vi "Autobalance Calculate One DOF.vi"(6 "Max Voltage":dbl, 8 "Autobalance Persistant Values In":T1, 10 "Error Tolerance":dbl) -> (0 "Autobalance Persistant Values Out":T1, 2 "Balanced Command":dbl)   [LabVIEW 2009]
uses:
  Autobalance Status Data.ctl
  Apps/Yes No Button.ctl
  Autobalance Stage.ctl
  Autobalance Data Point.ctl
  Course2MediumTransition.ctl
panel:
  # "Cmd"
  # "Servo"
  # "Cmd"
  # "Servo"
  # "Cmd"
  # "Servo"
  # "Cmd"
  # "Servo"
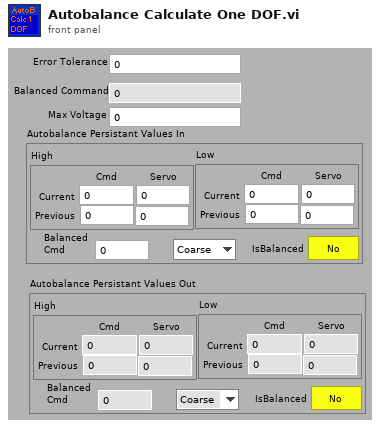
[diagram p1: front panel]
types:
  T1 = typedef "Autobalance Status Data.ctl" = cluster{"IsBalanced":T2, "Autobalance Stage":T3, "High":T4, "Low":T4, "Balanced \nCmd":dbl}
  T2 = typedef "Yes No Button.ctl" = bool
  T3 = typedef "Autobalance Stage.ctl" = enum16{"Coarse", "Fine", "Done"}
  T4 = typedef "Autobalance Data Point.ctl" = cluster{"cCmd":dbl, "cServo":dbl, "pCmd":dbl, "pServo":dbl}
  T5 = typedef "Course2MediumTransition.ctl" = enum16{"High Changed", "Low Changed", "Both Changed", "None Changed"}
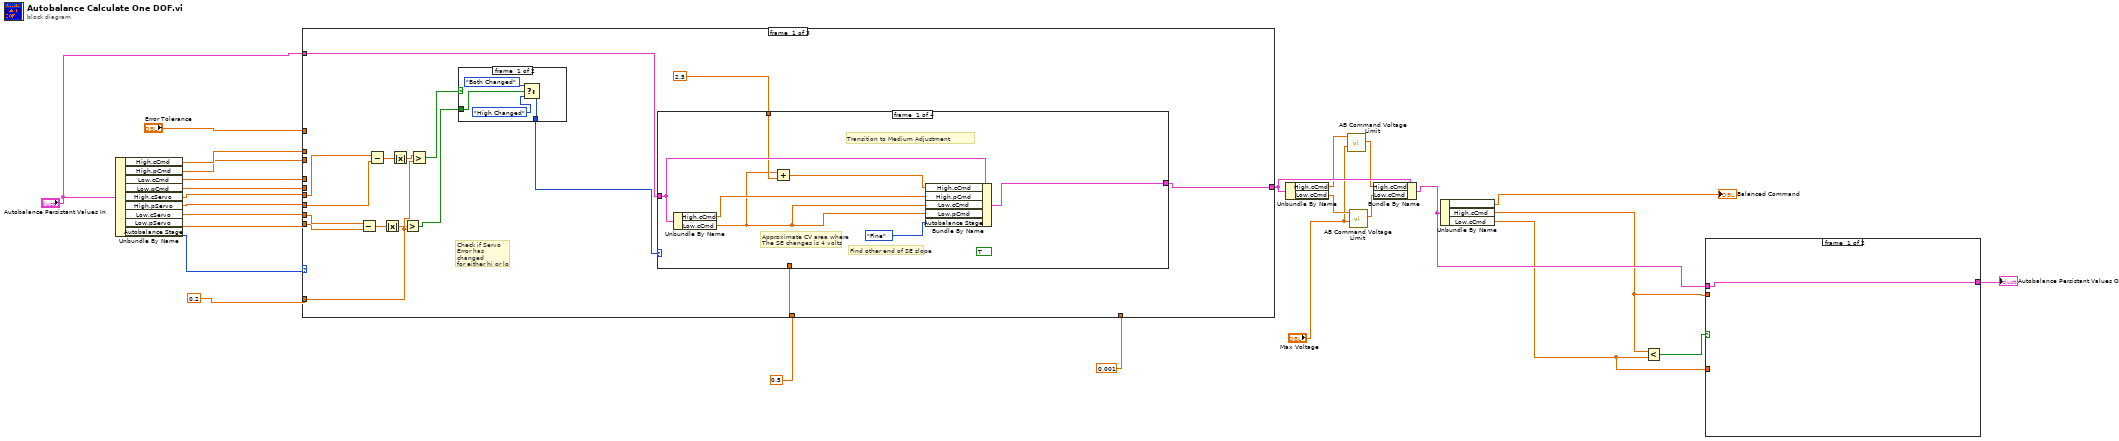
[diagram p0: block diagram]
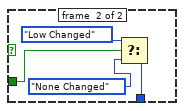
[diagram p2: hidden frame]
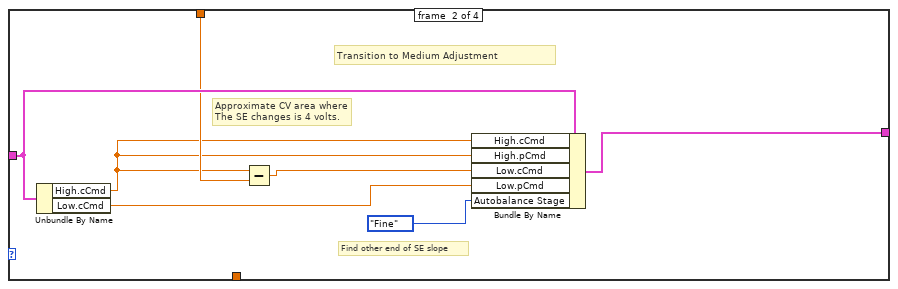
[diagram p3: hidden frame]
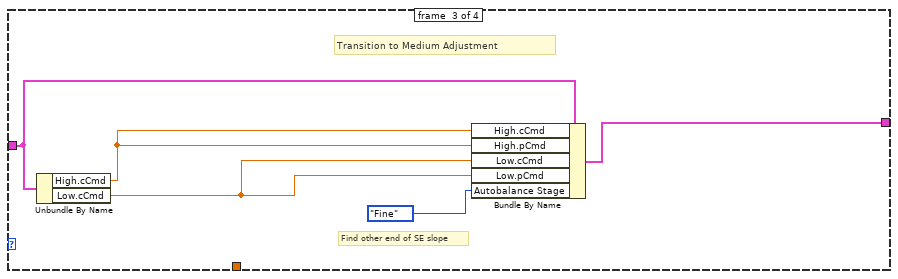
[diagram p4: hidden frame]
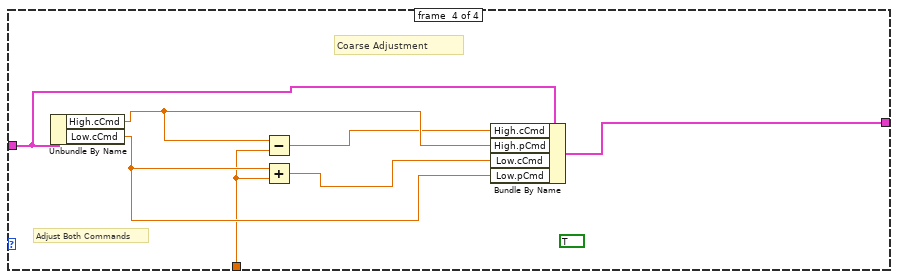
[diagram p5: hidden frame]
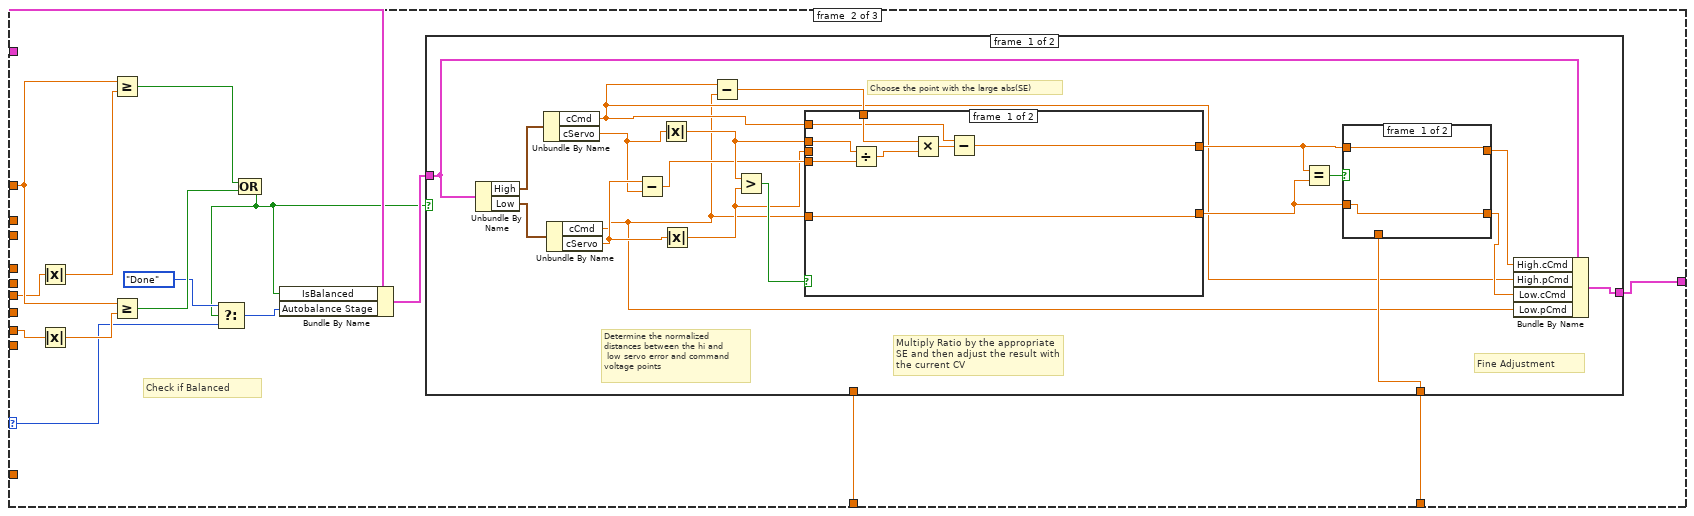
[diagram p6: hidden frame]
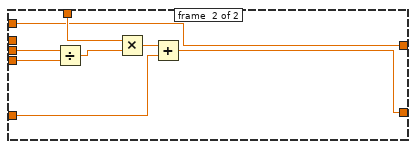
[diagram p7: hidden frame]
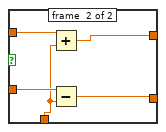
[diagram p8: hidden frame]
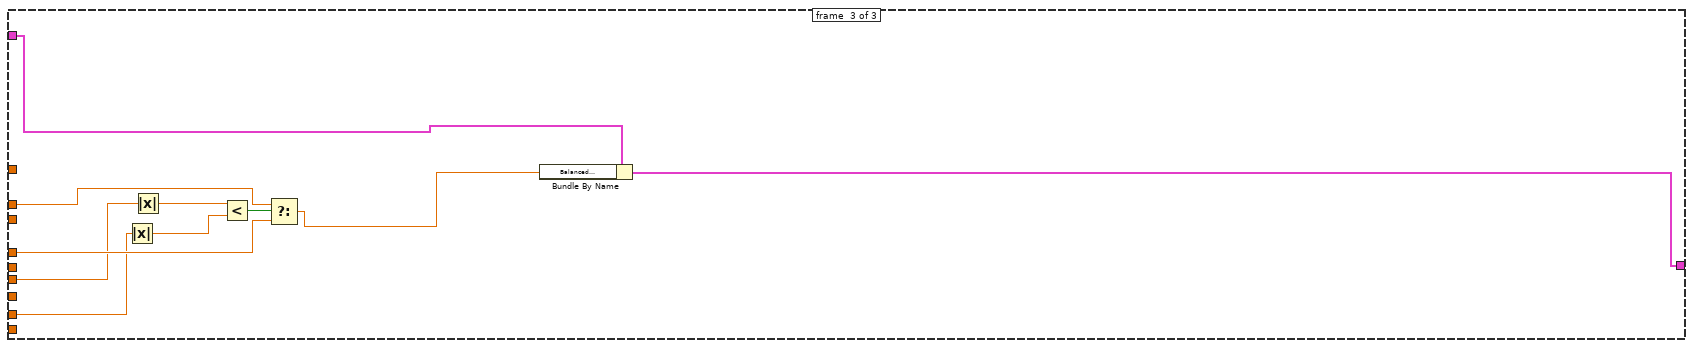
[diagram p10: hidden frame]
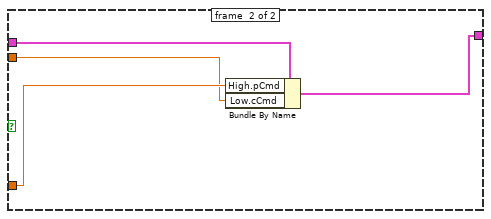
[diagram p11: hidden frame]
diagram:
  n1 = Unbundle By Name("Autobalance Persistant Values In") -> ("High.cCmd"=w17:dbl, "High.pCmd"=w16:dbl, "Low.cCmd"=w15:dbl, "Low.pCmd"=w14:dbl, "High.cServo"=w26:dbl, "High.pServo"=w25:dbl, "Low.cServo"=w24:dbl, "Low.pServo"=w23:dbl, "Autobalance Stage"=w22:T3)
  n2 = case shown="\"Fine\"" w22 {
    selector: w22 -> [_ w87 _]
    tunnel: w26 -> [w41 w81 w140]
    tunnel: w25 -> [w42 _ _]
    tunnel: w24 -> [w40 w80 w139]
    tunnel: w23 -> [w39 _ _]
    tunnel: "Autobalance Persistant Values In" -> [w28 w88 w138]
    tunnel: [w36 w83 w136] -> w6
    tunnel: "Error Tolerance" -> [_ w85 _]
    tunnel: 0.2 -> [w38 _ _]
    tunnel: 0.5 -> [w37 w78 _]
    tunnel: w17 -> [_ _ w142]
    tunnel: w16 -> [_ _ _]
    tunnel: w15 -> [_ _ w141]
    tunnel: w14 -> [_ _ _]
    tunnel: 0.001 -> [_ w77 _]
    frame #0 {
      # "Check if Servo \nError has changed\nfor either hi or lo"
      n3 = Subtract(x=w40, y=w39) -> (x-y=w33:dbl)
      n4 = Subtract(x=w41, y=w42) -> (x-y=w35:dbl)
      n5 = Absolute Value(x=w33) -> (abs(x)=w32:dbl)
      n6 = Absolute Value(x=w35) -> (abs(x)=w34:dbl)
      n7 = Greater?(x=w32, y=w38) -> (0:w30:bool)
      n8 = Greater?(x=w34, y=w38) -> (0:w31:bool)
      n9 = case shown="True" w31 {
        tunnel: w30 -> [w46 w50]
        tunnel: [w43 w47] -> w29
        frame #0 {
          n10 = Select(t=Course2MediumTransition."Both Changed", s=w46, f=Course2MediumTransition."High Changed" ("Course2MediumTransition")) -> (s? t:f=w43:T5)
        }
        frame #1 {
          n11 = Select(t=Course2MediumTransition."Low Changed", s=w50, f=Course2MediumTransition."None Changed" ("Course2MediumTransition")) -> (s? t:f=w47:T5)
        }
      }
      n12 = case shown="\"High Changed\"" w29 {
        tunnel: w28 -> [w57 w64 w69 w76]
        tunnel: [w56 w63 w68 w75] -> w36
        tunnel: w37 -> [_ _ _ w72]
        tunnel: 2.5 -> [w54 w59 _ _]
        frame #0 {
          (unwired) TRUE
          # "Approximate CV area where\nThe SE changes is 4 volts"
          # "Transition to Medium Adjustment"
          # "Find other end of SE slope"
          n13 = Unbundle By Name(w57) -> ("High.cCmd"=w53:dbl, "Low.cCmd"=w51:dbl)
          n14 = Add(x=w51, y=w54) -> (x+y=w52:dbl)
          n15 = Bundle By Name(cluster=w57, "High.cCmd"=w52, "High.pCmd"=w53, "Low.cCmd"=w51, "Low.pCmd"=w51, "Autobalance Stage"=Autobalance_Stage."Fine" ("t")) -> (w56:T1)
        }
        frame #1 {
          # "Approximate CV area where\nThe SE changes is 4 volts."
          # "Transition to Medium Adjustment"
          # "Find other end of SE slope"
          n16 = Unbundle By Name(w64) -> ("High.cCmd"=w58:dbl, "Low.cCmd"=w61:dbl)
          n17 = Subtract(x=w58, y=w59) -> (x-y=w60:dbl)
          n18 = Bundle By Name(cluster=w64, "High.cCmd"=w58, "High.pCmd"=w58, "Low.cCmd"=w60, "Low.pCmd"=w61, "Autobalance Stage"=Autobalance_Stage."Fine" ("t")) -> (w63:T1)
        }
        frame #2 {
          # "Transition to Medium Adjustment"
          # "Find other end of SE slope"
          n19 = Unbundle By Name(w69) -> ("High.cCmd"=w66:dbl, "Low.cCmd"=w65:dbl)
          n20 = Bundle By Name(cluster=w69, "High.cCmd"=w66, "High.pCmd"=w66, "Low.cCmd"=w65, "Low.pCmd"=w65, "Autobalance Stage"=Autobalance_Stage."Fine" ("t")) -> (w68:T1)
        }
        frame #3 {
          (unwired) TRUE
          # "Coarse Adjustment"
          # "Adjust Both Commands"
          n21 = Unbundle By Name(w76) -> ("High.cCmd"=w74:dbl, "Low.cCmd"=w73:dbl)
          n22 = Subtract(x=w74, y=w72) -> (x-y=w71:dbl)
          n23 = Add(x=w73, y=w72) -> (x+y=w70:dbl)
          n24 = Bundle By Name(cluster=w76, "High.cCmd"=w71, "High.pCmd"=w74, "Low.cCmd"=w70, "Low.pCmd"=w73) -> (w75:T1)
        }
      }
    }
    frame #1 {
      # "Check if Balanced"
      n25 = Absolute Value(x=w81) -> (abs(x)=w89:dbl)
      n26 = Absolute Value(x=w80) -> (abs(x)=w90:dbl)
      n27 = Greater Or Equal?(x=w85, y=w89) -> (x >= y?=w91:bool)
      n28 = Greater Or Equal?(x=w85, y=w90) -> (x >= y?=w92:bool)
      n29 = Compound Arithmetic op=OR(w91, w92) -> (w82:bool)
      n30 = Select(t=Autobalance_Stage."Done", s=w82, f=w87) -> (s? t:f=w79:T3)
      n31 = Bundle By Name(cluster=w88, "IsBalanced"=w82, "Autobalance Stage"=w79) -> (w84:T1)
      n32 = case shown="False" w82 {
        tunnel: w84 -> [w109 w135]
        tunnel: [w108 w135] -> w83
        tunnel: w78 -> [_ _]
        tunnel: w77 -> [w106 _]
        frame #0 {
          # "Choose the point with the large abs(SE)"
          # "Multiply Ratio by the appropriate\nSE and then adjust the result with \nthe current CV"
          # "Determine the normalized \ndistances between the hi and\n low servo error and command\nvoltage points"
          # "Fine Adjustment"
          n33 = Unbundle By Name(w109) -> ("High"=w111:T4, "Low"=w110:T4)
          n34 = Unbundle By Name(w111) -> ("cCmd"=w94:dbl, "cServo"=w102:dbl)
          n35 = Unbundle By Name(w110) -> ("cCmd"=w93:dbl, "cServo"=w103:dbl)
          n36 = Subtract(x=w103, y=w102) -> (x-y=w99:dbl)
          n37 = Absolute Value(x=w102) -> (abs(x)=w100:dbl)
          n38 = Absolute Value(x=w103) -> (abs(x)=w95:dbl)
          n39 = Subtract(x=w94, y=w93) -> (x-y=w98:dbl)
          n40 = Greater?(x=w100, y=w95) -> (0:w101:bool)
          n41 = case shown="True" w101 {
            tunnel: w100 -> [w119 _]
            tunnel: w99 -> [w118 w127]
            tunnel: w98 -> [w116 w125]
            tunnel: w93 -> [w115 w123]
            tunnel: [w115 w120] -> w97
            tunnel: [w114 w121] -> w96
            tunnel: w95 -> [_ w122]
            tunnel: w94 -> [w112 w121]
            frame #0 {
              n42 = Divide(x=w119, y=w118) -> (x/y=w117:dbl)
              n43 = Multiply(x=w116, y=w117) -> (x*y=w113:dbl)
              n44 = Subtract(x=w112, y=w113) -> (x-y=w114:dbl)
            }
            frame #1 {
              n45 = Divide(x=w122, y=w127) -> (x/y=w126:dbl)
              n46 = Multiply(x=w125, y=w126) -> (x*y=w124:dbl)
              n47 = Add(x=w124, y=w123) -> (x+y=w120:dbl)
            }
          }
          n48 = Equal?(x=w96, y=w97) -> (x = y?=w107:bool)
          n49 = case shown="True" w107 {
            tunnel: w96 -> [w129 w132]
            tunnel: w97 -> [w128 w134]
            tunnel: w106 -> [_ w133]
            tunnel: [w129 w131] -> w105
            tunnel: [w128 w130] -> w104
            frame #0 {
            }
            frame #1 {
              n50 = Add(x=w132, y=w133) -> (x+y=w131:dbl)
              n51 = Subtract(x=w134, y=w133) -> (x-y=w130:dbl)
            }
          }
          n52 = Bundle By Name(cluster=w109, "High.cCmd"=w105, "High.pCmd"=w94, "Low.cCmd"=w104, "Low.pCmd"=w93) -> (w108:T1)
        }
        frame #1 {
        }
      }
    }
    frame #2 {
      n53 = Absolute Value(x=w139) -> (abs(x)=w144:dbl)
      n54 = Absolute Value(x=w140) -> (abs(x)=w143:dbl)
      n55 = Less?(x=w143, y=w144) -> (x < y?=w145:bool)
      n56 = Select(t=w142, s=w145, f=w141) -> (s? t:f=w137:dbl)
      n57 = Bundle By Name(cluster=w138, "Balanced \nCmd"=w137) -> (w136:T1)
    }
  }
  n58 = Unbundle By Name(w6) -> ("High.cCmd"=w5:dbl, "Low.cCmd"=w3:dbl)
  n59 = call "AB Command Voltage Limit.vi"("Max Voltage"="Max Voltage", "Command In"=w5) -> ("Command Out"=w4:dbl)  [unwired: 9 out]
  n60 = call "AB Command Voltage Limit.vi"("Max Voltage"="Max Voltage", "Command In"=w3) -> ("Command Out"=w2:dbl)  [unwired: 9 out]
  n61 = Bundle By Name(cluster=w6, "High.cCmd"=w4, "Low.cCmd"=w2) -> (w12:T1)
  n62 = Unbundle By Name(w12) -> ("Balanced \nCmd"=→"Balanced Command":dbl, "High.cCmd"=w11:dbl, "Low.cCmd"=w10:dbl)
  n63 = Less?(x=w11, y=w10) -> (x < y?=w13:bool)
  n64 = case shown="True" w13 {
    tunnel: w12 -> [w146 w150]
    tunnel: [w146 w149] -> w9
    tunnel: w11 -> [_ w147]
    tunnel: w10 -> [_ w148]
    frame #0 {
    }
    frame #1 {
      n65 = Bundle By Name(cluster=w150, "High.pCmd"=w148, "Low.cCmd"=w147) -> (w149:T1)
    }
  }
  "Autobalance Persistant Values Out" <- w9
